vi "PixyCam_BuildTarget.vi"(3 "RawData":u16[](array[numeric])) -> (0 "Target":T1 {"Angle" format="%x"; "Height" format="%x"; "Width" format="%x"; "Y Center" format="%x"; "X Center" format="%x"; "Signature Number" format="%x"; "Checksum" format="%x"; "Target Type" items=["PIXY_START_WORD"=43605, "PIXY_START_WORD_CC"=43606, "PIXY_START_WORDX"=21930]}, 1 "Valid Checksum":bool)   [LabVIEW 2016, in "PixyCam_LabVIEW.lvlib"]
uses:
  PixyCam_LabVIEW.lvlib
  PixyCam_TargetData.ctl
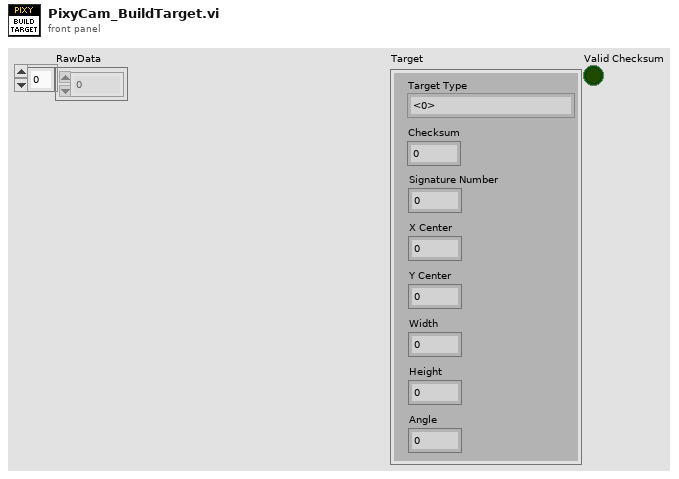
[diagram p1: front panel]
types:
  T1 = typedef "PixyCam_LabVIEW.lvlib/PixyCam_TargetData.ctl" = cluster{"Target Type":u16, "Checksum":u16, "Signature Number":u16, "X Center":u16, "Y Center":u16, "Width":u16, "Height":u16, "Angle":u16}
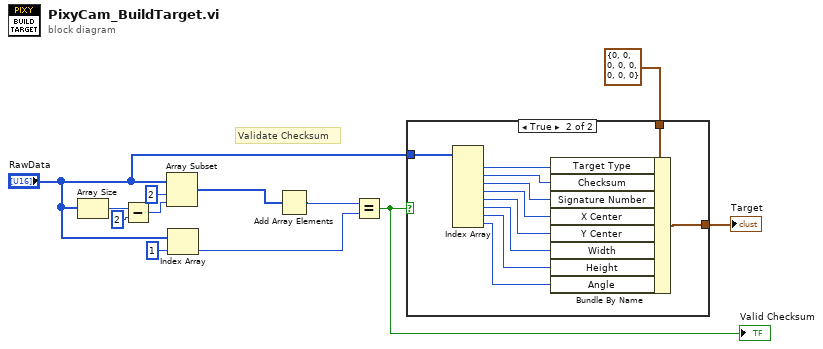
[diagram p0: block diagram]
diagram:
  # "Validate Checksum"
  n1 = Array Size(array="RawData") -> (size(s)=w6:i32)
  n2 = Subtract(x=w6, y=2) -> (x-y=w4:i32)
  n3 = Array Subset(array="RawData", index=2, length=w4) -> (w2:u16[])
  n4 = Index Array(array="RawData", index=1) -> (element=w10:u16)
  n5 = Add Array Elements(numeric array=w2) -> (sum=w1:u16)
  n6 = Equal?(x=w1, y=w10) -> (x = y?=w9:bool)
  "Valid Checksum" <- w9
  n7 = case shown="True" w9 {
    tunnel: [w13 w24] -> w8
    tunnel: T1 {"Target Type"=0, "Checksum"=0, "Signature Number"=0, "X Center"=0, "Y Center"=0, "Width"=0, "Height"=0, "Angle"=0} ("Target 2") -> [w13 w23]
    tunnel: "RawData" -> [_ w22]
    frame False {
      # "Return empty target if checksum fails"
    }
    frame True {
      n8 = Index Array(array=w22) -> (element #1=w21:u16, element #2=w20:u16, element #3=w19:u16, element #4=w18:u16, element #5=w17:u16, element #6=w16:u16, element #7=w15:u16, element #8=w14:u16)  [unwired: 8 in]
      n9 = Bundle By Name(cluster=w23, "Target Type"=w21, "Checksum"=w20, "Signature Number"=w19, "X Center"=w18, "Y Center"=w17, "Width"=w16, "Height"=w15, "Angle"=w14) -> (w24:T1)
    }
  }
  "Target" <- w8
